vi "Very_Simple_Calculator.vi"() -> ()   [LabVIEW 2010]
panel:
  in  "stop":bool
  out "X / Y":dbl
  out "X * Y":dbl
  out "X - Y":dbl
  out "X + Y":dbl
  in  "Y":dbl
  in  "X":dbl
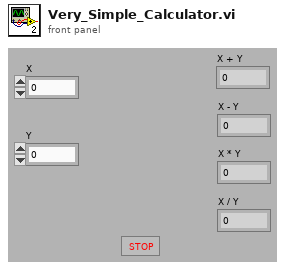
[diagram p1: front panel]
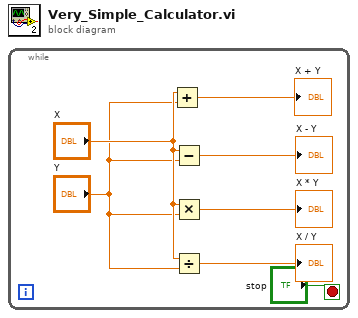
[diagram p0: block diagram]
diagram:
  n1 = while {
    stop <- "stop" stop-if-true
    n2 = Add(x="X", y="Y") -> (x+y=→"X + Y":dbl)
    n3 = Subtract(x="X", y="Y") -> (x-y=→"X - Y":dbl)
    n4 = Multiply(x="X", y="Y") -> (x*y=→"X * Y":dbl)
    n5 = Divide(x="X", y="Y") -> (x/y=→"X / Y":dbl)
  }
